vi "marshalling.vi"(8 "error in (no error)":errorcluster, 10 "Variant":variant, 11 "Serializer in":refnum<class "Serializer.lvclass">) -> (0 "error out":errorcluster, 2 "String":string, 3 "Serializer out":refnum<class "Serializer.lvclass">)   [LabVIEW 2013, in "Serializer.lvclass"]
uses:
  Serializer.lvclass
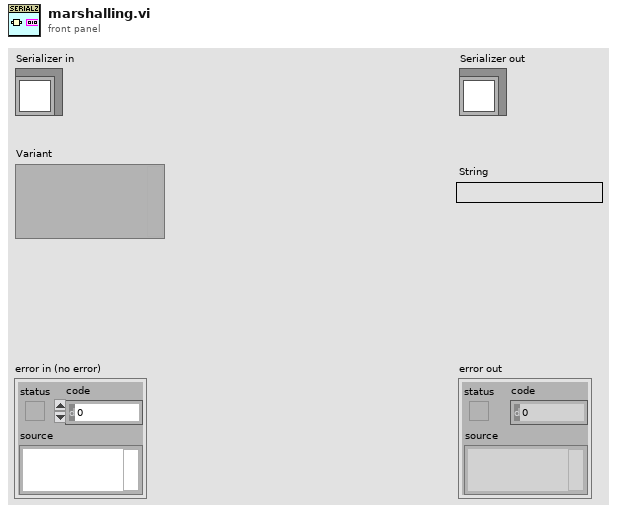
[diagram p1: front panel]
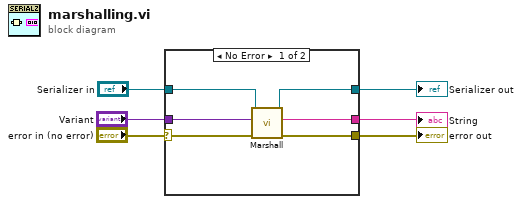
[diagram p0: block diagram]
diagram:
  n1 = case shown="No Error" "error in (no error)" {
    selector: "error in (no error)" -> [w8 w14]
    tunnel: [w7 w14] -> w5
    tunnel: [w9 w13] -> w3
    tunnel: "Serializer in" -> [w10 w13]
    tunnel: "Variant" -> [w12 _]
    tunnel: [w11 _] -> w1
    frame No Error {
      n2 = call "Marshall.vi"("error in (no error)"=w8, "Variant"=w12, "Serializer in"=w10) -> ("error out"=w7:errorcluster, "String"=w11:string, "Serializer out"=w9:refnum<class "Serializer.lvclass">)  [unwired: 6 in]
    }
    frame Error {
    }
  }
  "error out" <- w5
  "Serializer out" <- w3
  "String" <- w1
